vi "Update Indecies.vi"(8 "error in (no error)":errorcluster, 11 "Column Data Type Definitions in":refnum<class "Generic Data Type.lvclass">[](array[class])) -> (0 "error out":errorcluster, 3 "Column Data Type Definitions out":refnum<class "Generic Data Type.lvclass">[](array[class]))   [LabVIEW 2018, in "DataGrid Config.lvclass"]
uses:
  DataGrid Config.lvclass
  Data Type Classes/Generic/Generic Data Type.lvclass
  Data Type Classes/Generic/Generic Data Type.lvclass/Generic Data Type.ctl
  Data Type Classes/Generic/Write Column Index.vi
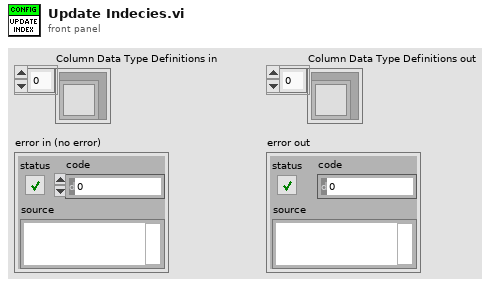
[diagram p1: front panel]
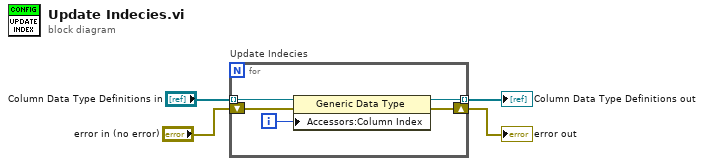
[diagram p0: block diagram]
diagram:
  n1 = for "Update Indecies" {
    tunnel: "Column Data Type Definitions in" -> [w9] mode=indexing
    tunnel: [w7] -> w2 mode=indexing
    shift-right: [w5] -> w4
    shift-left: "error in (no error)" -> [w6]
    i -> [w8]
    n2 = property class="Generic Data Type"(reference=w9, error in=w6, "Accessors:Column Index"=w8) -> (reference out=w7:refnum<class "Generic Data Type.lvclass">, error out=w5:errorcluster)
  }
  "error out" <- w4
  "Column Data Type Definitions out" <- w2
